vi "Transfer CAN Logs.vi"(6 "address":string, 7 "Destination":path, 8 "error in (no error)":errorcluster, 11 "Raw CAN Log files":string[](array[string])) -> (0 "error out":errorcluster, 2 "Files moved":path[](array[path]))   [LabVIEW 2010, in "CAN Log Transfer and Convert.lvlib"]
uses:
  CAN Log Transfer and Convert.lvlib
  <vilib>/addons/internet/NI_InternetTK_FTP_VIs.lvlib
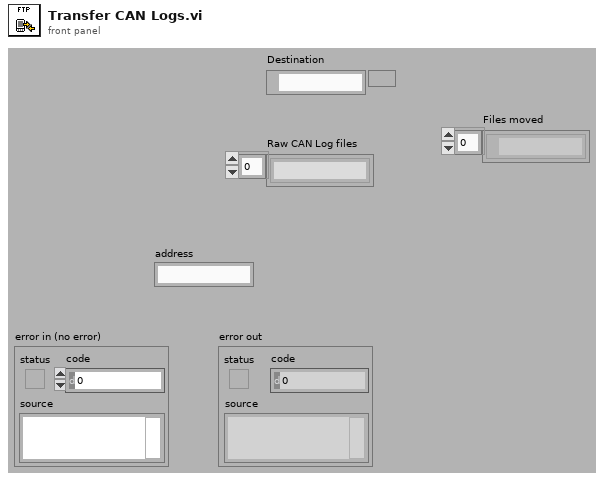
[diagram p1: front panel]
types:
  T1 = cluster{"remote path":string, "local path":path, "binary":bool}
  T2 = typedef "FTP Session.ctl" = refnum<k1>
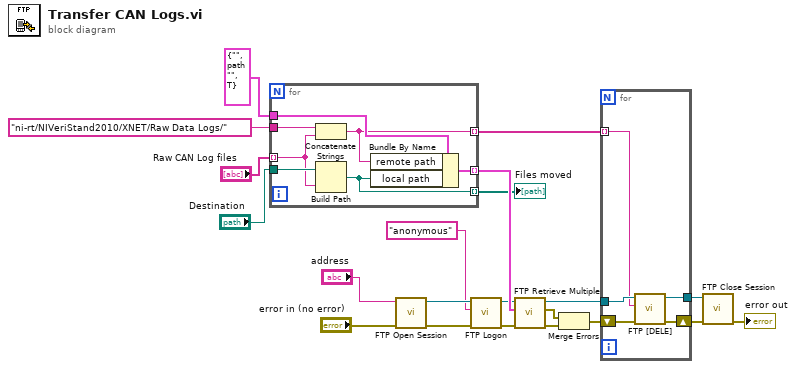
[diagram p0: block diagram]
diagram:
  n1 = for {
    tunnel: T1 {"remote path"="", "local path"=path "", "binary"=TRUE} ("transfer spec") -> [w28]
    tunnel: "Destination" -> [w27]
    tunnel: "ni-rt/NIVeriStand2010/XNET/Raw Data Logs/" -> [w26]
    tunnel: "Raw CAN Log files" -> [w25] mode=indexing
    tunnel: [w24] -> w17 mode=indexing
    tunnel: [w23] -> w14 mode=indexing
    tunnel: [w22] -> w11 mode=indexing
    n2 = Concatenate Strings(w26, w25) -> (w22:string)
    n3 = Build Path(base path=w27, name or relative path=w25) -> (appended path=w23:path)
    n4 = Bundle By Name(cluster=w28, "remote path"=w22, "local path"=w23) -> (w24:T1)
  }
  "Files moved" <- w14
  n5 = call <vilib>:"FTP Open Session.vi"("error in (no error)"="error in (no error)", "address"="address") -> ("error out"=w10:errorcluster, "ftp session"=w9:T2)  [unwired: 6 in, 2 out]
  n6 = call <vilib>:"FTP Logon.vi"("error in (no error)"=w10, "user"="anonymous", "ftp session"=w9) -> ("error out"=w5:errorcluster, "ftp session out"=w4:T2)  [unwired: 5 in, 2 out]
  n7 = call <vilib>:"FTP Retrieve Multiple.vi"("error in (no error)"=w5, "file specifications"=w17, "ftp session"=w4) -> ("error out"=w16:errorcluster, "file errors"=w15:errorcluster[], "ftp session out"=w12:T2)  [unwired: 5 in, 1 out]
  n8 = Merge Errors(w15, w16) -> (w13:errorcluster)
  n9 = for {
    tunnel: w12 -> [w32]
    tunnel: w11 -> [w31] mode=indexing
    shift-right: [w30] -> w2
    shift-left: w13 -> [w33]
    tunnel: [w29] -> w3
    n10 = call <vilib>:"FTP [DELE].vi"("error in (no error)"=w33, "file path"=w31, "ftp session"=w32) -> ("error out"=w30:errorcluster, "ftp session out"=w29:T2)  [unwired: 5 in, 2 out]
  }
  n11 = call <vilib>:"FTP Close Session.vi"("error in (no error)"=w2, "ftp session"=w3) -> ("error out"=→"error out":errorcluster)  [unwired: 6 in, 3 out]
